vi "No File Loaded Message.vi"() -> (0 "no file loaded string":string)   [LabVIEW 2017]
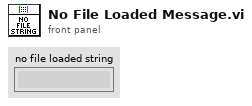
[diagram p1: front panel]
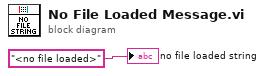
[diagram p0: block diagram]
diagram:
  "no file loaded string" <- "<no file loaded>" ("Front Panel Window:Title")
